vi "Copy-Exchange Trace.vi"(7 "Trace2 (2: Trace 2)":i32(ring)=2 items=["Trace 1"=1, "Trace 2"=2, "Trace 3"=3, "Trace 4"=4, "Trace 5"=5, "Trace 6"=6], 8 "error in (no error)":errorcluster, 9 "Trace1 (1: Trace 1)":i32(ring)=1 items=["Trace 1"=1, "Trace 2"=2, "Trace 3"=3, "Trace 4"=4, "Trace 5"=5, "Trace 6"=6], 10 "Operation (0: Copy)":i32(ring) items=["Copy", "Exchange"], 11 "VISA resource name":refnum<visa-resource-name>) -> (0 "error out":errorcluster, 3 "VISA resource name out":refnum<visa-resource-name>)   [LabVIEW 2014, in "Agilent MXA Series.lvlib"]
doc: "Copies or Exchanges the selected traces."
uses:
  Agilent MXA Series.lvlib
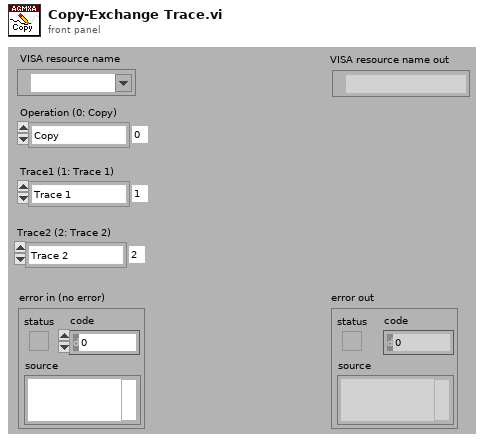
[diagram p1: front panel]
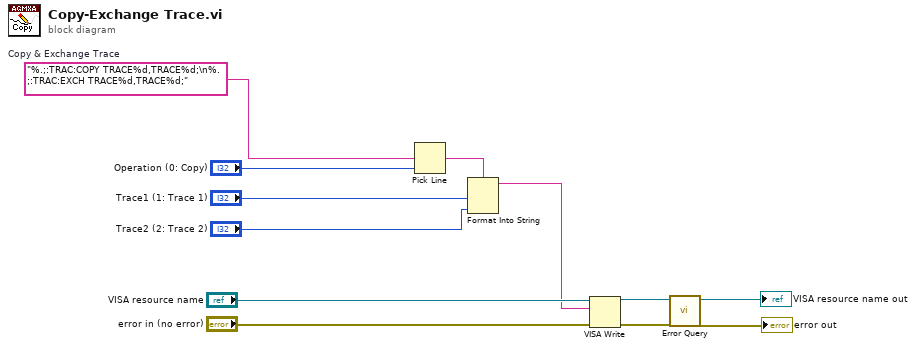
[diagram p0: block diagram]
diagram:
  w3 = "%.;:TRAC:COPY TRACE%d,TRACE%d;\n%.;:TRAC:EXCH TRACE%d,TRACE%d;"  # Copy & Exchange Trace
  n1 = Pick Line(multi-line string=w3, line index="Operation (0: Copy)") -> (output string=w2:string)  [unwired: 1 in]
  n2 = Format Into String(format string=w2, "Trace1 (1: Trace 1)", "Trace2 (2: Trace 2)") -> (resulting string=w8:string)  [unwired: 2 in, 1 out]
  n3 = VISA Write(VISA resource name="VISA resource name", write buffer=w8, error in (no error)="error in (no error)") -> (VISA resource name out=w7:refnum<visa-resource-name>, error out=w6:errorcluster)  [unwired: 1 out]
  n4 = call "Error Query.vi"("error in (no error)"=w6, "VISA resource name"=w7) -> ("error out"=→"error out":errorcluster, "VISA resource name out"=→"VISA resource name out":refnum<visa-resource-name>)  [unwired: 6 in, 2 out]
